vi "IDD Test Configure SMU.vi"(6 "script name":string="IDD", 7 "SMU Settings":T2={"Level"=1.8, "Level Range"=6.0, "Limit"=0.01, "Limit Range"=0.01, "Sense"=1008} {"Sense" items=["Local"=1008, "Remote"=1009]}, 8 "error in (no error)":errorcluster, 9 "Publishable IDs":string[](array[string])=["IDD_LowPower", "IDD_DVC_Cmin", "IDD_DVC_Cmax"], 10 "Pins":string[](array[string])=["VDD"], 11 "Semiconductor Module Context":T3) -> (0 "error out":errorcluster)   [LabVIEW 2013]
uses:
  <vilib>/NI_TestStand_SemiconductorModule/NI_TestStand_Semiconductor_Module.lvlibp/PinMap/General/SemiconductorModuleContext.ctl
  <instrlib>/niDCPower/nidcpower.llb/niDCPower Sense.ctl
  <instrlib>/niHSDIO/niHSDIO.llb/niHSDIO_ctl Trigger Script - trigID Values (Ring).ctl
  <vilib>/NI_TestStand_SemiconductorModule/NI_TestStand_Semiconductor_Module.lvlibp/PinMap/DC Power/PinsToNIDCPowerSessions.vi
  <vilib>/NI_TestStand_SemiconductorModule/NI_TestStand_Semiconductor_Module.lvlibp/PinMap/General/Publish/PublishDataDouble2D.vi
  <vilib>/NI_TestStand_SemiconductorModule/NI_TestStand_Semiconductor_Module.lvlibp
panel:
  out "current measurements":dbl[][](array[numeric])
  out "State":string
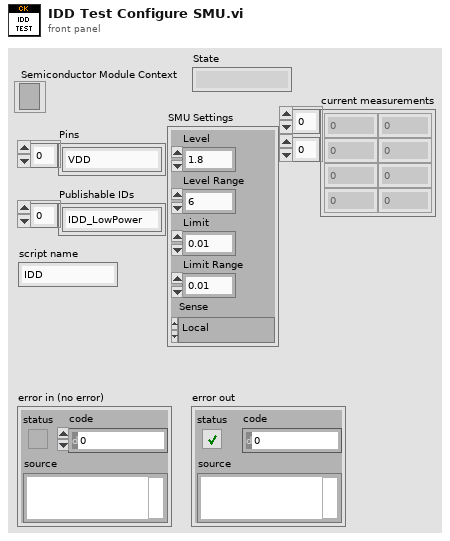
[diagram p1: front panel]
types:
  T1 = typedef "niDCPower Sense.ctl" = i32
  T2 = cluster{"Level":dbl, "Level Range":dbl, "Limit":dbl, "Limit Range":dbl, "Sense":T1}
  T3 = typedef "NI_TestStand_Semiconductor_Module.lvlibp/SemiconductorModuleContext.ctl" = refnum<k7>
  T4 = typedef "niHSDIO_ctl Trigger Script - trigID Values (Ring).ctl" = string
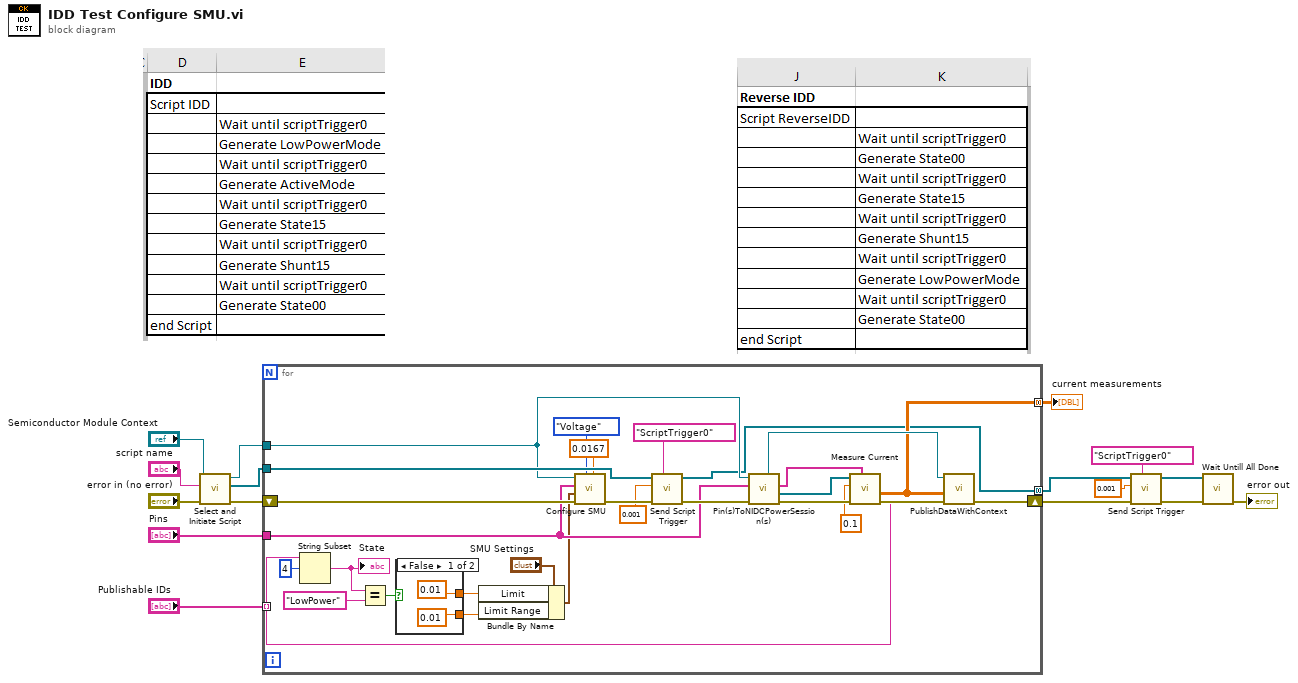
[diagram p0: block diagram]
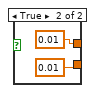
[diagram p2: hidden frame]
diagram:
  n1 = call "Select and Initiate Script.vi"("error in (no error)"="error in (no error)", "script name"="script name", "Semiconductor Module Context"="Semiconductor Module Context") -> ("error out"=w10:errorcluster, "HSDIO GEN Sessions Out"=w8:refnum<k15>[], "Semiconductor Module Context Out"=w14:T3)  [unwired: 6 in]
  n2 = for {
    tunnel: "Pins" -> [w32]
    tunnel: w14 -> [w33]
    tunnel: w8 -> [w39]
    tunnel: "Publishable IDs" -> [w29] mode=indexing
    shift-right: [w38] -> w6
    shift-left: w10 -> [w35]
    tunnel: [w18] -> w9 mode=concatenating
    tunnel: [w17] -> w4 mode=concatenating
    n3 = String Subset(string=w29, offset (0)=4) -> (substring=w27:string)  [unwired: 1 in]
    "State" <- w27
    n4 = Equal?(x=w27, y="LowPower" ("regular expression")) -> (x = y?=w25:bool)
    n5 = case shown="False" w25 {
      tunnel: [0.01 ("Limit") 0.01 ("Limit")] -> w24
      tunnel: [0.01 ("Limit Range") 0.01 ("Limit Range")] -> w23
      frame False {
      }
      frame True {
      }
    }
    n6 = Bundle By Name(cluster="SMU Settings", "Limit"=w24, "Limit Range"=w23) -> (w30:T2)
    n7 = call "Configure SMU.vi"("aperture time"=0.0167, "Source Mode"=enum16{"Voltage", "Current"}."Voltage", "error in (no error)"=w35, "Settings"=w30, "Pins"=w32, "Semiconductor Module Context"=w33) -> ("error out"=w34:errorcluster)  [unwired: 5 in]
    n8 = call "Send Script Trigger.vi"("trigger id (script trigger 0)"=T4 "ScriptTrigger0", "error in (no error)"=w34, "Delay Time (s)"=0.001, "HSDIO Sessions In"=w39) -> ("error out"=w36:errorcluster, "HSDIO Sessions Out"=w17:refnum<k15>[])  [unwired: 6 in]
    n9 = call-poly <vilib>:"Pin(s)ToNIDCPowerSession(s).vi"("error in (no error)"=w36, "Pins"=w32, "Semiconductor Module Context"=w33) -> ("error out"=w40:errorcluster, "Instrument Sessions"=w44:refnum<k15>[], "Channel Lists"=w42:string[], "Pin Query Context"=w41:refnum<class "MultiplePinMultipleSessionQueryContext.lvclass">)  [unwired: 4 in, 1 out]
    n10 = call "Measure Current.vi"("Channel Lists"=w42, "error in (no error)"=w40, "Delay Time (s)"=0.1, "DCPower Sessions In"=w44) -> ("error out"=w43:errorcluster, "current measurements"=w18:dbl[][])  [unwired: 5 in, 1 out]
    n11 = call-poly <vilib>:"PublishDataWithContext.vi"("Published Data Id"=w29, "error in (no error)"=w43, "Data In"=w18, "Pin Query Context"=w41) -> ("error out"=w38:errorcluster)  [unwired: 6 in, 1 out]
  }
  "current measurements" <- w9
  n12 = call "Send Script Trigger.vi"("trigger id (script trigger 0)"=T4 "ScriptTrigger0", "error in (no error)"=w6, "Delay Time (s)"=0.001, "HSDIO Sessions In"=w4) -> ("error out"=w5:errorcluster, "HSDIO Sessions Out"=w1:refnum<k15>[])  [unwired: 6 in]
  n13 = call "Wait Untill All Done.vi"("error in (no error)"=w5, "HSDIO Sessions In"=w1) -> ("error out"=→"error out":errorcluster)  [unwired: 8 in, 1 out]
